vi "Read_resistance.vi"() -> ()   [LabVIEW 2017]
uses:
  <instrlib>/Agilent B2900 Series/Public/Configure/Measurement/Configure Measurement (Resistance).vi
  <instrlib>/Agilent B2900 Series/Public/Data/Read Measurement Result (Single Point).vi
  <instrlib>/Agilent B2900 Series/Agilent B2900 Series.lvlib
panel:
  out "Measurement Result":dbl
  in  "Data Mode (5: Voltage)":i32(ring)=5 items=["Current", "Resistance", "Source Output Setting", "Status", "Time", "Voltage"]
  in  "Resistance Range Lower Limit (2 Ohm)":dbl=2.0
  in  "Resistance Range Upper Limit (2E+8 Ohm)":dbl=200000000.0
  in  "Resistance NPLC (0.1)":dbl=0.1
  in  "Resistance Measurement Mode (1: Auto)":i32(ring)=1 items=["Manual", "Auto"]
  in  "Resistance Range (2 Ohm)":dbl=2.0
  in  "VISA resource name":refnum<visa-resource-name>
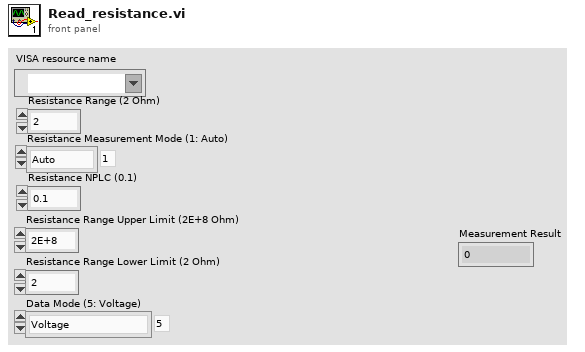
[diagram p1: front panel]
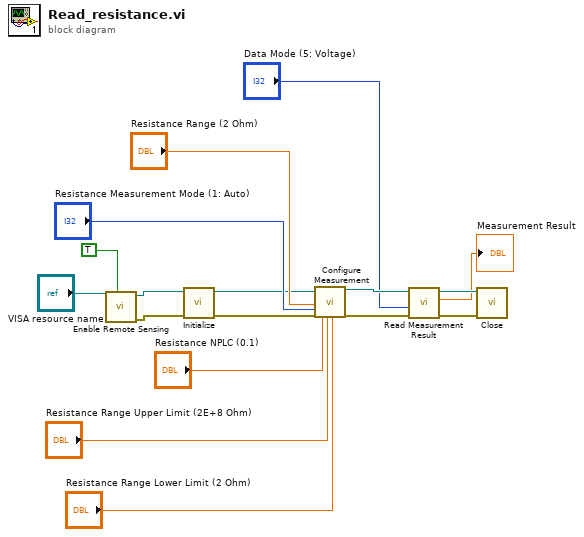
[diagram p0: block diagram]
diagram:
  n1 = call <instrlib>:"Enable Remote Sensing.vi"("Enable Remote Sensing (F: Disable)"=TRUE, "VISA resource name"="VISA resource name") -> ("error out"=w3:errorcluster, "VISA resource name out"=w1:refnum<visa-resource-name>)  [unwired: 8 in]
  n2 = call <instrlib>:"Initialize.vi"("error in (no error)"=w3, "VISA resource name"=w1) -> ("error out"=w5:errorcluster, "VISA resource name out"=w6:refnum<visa-resource-name>)  [unwired: 8 in]
  n3 = call-poly <instrlib>:"Configure Measurement.vi"("VISA resource name"=w6, "Resistance Range (2 Ohm)"="Resistance Range (2 Ohm)", "Resistance Measurement Mode (1: Auto)"="Resistance Measurement Mode (1: Auto)", "error in (no error)"=w5, "Resistance NPLC (0.1)"="Resistance NPLC (0.1)", "Resistance Range Upper Limit (2E+8 Ohm)"="Resistance Range Upper Limit (2E+8 Ohm)", "Resistance Range Lower Limit (2 Ohm)"="Resistance Range Lower Limit (2 Ohm)") -> ("VISA resource name out"=w12:refnum<visa-resource-name>, "error out"=w10:errorcluster)  [unwired: 11 in]
  n4 = call-poly <instrlib>:"Read Measurement Result.vi"("error in (no error)"=w10, "Data Mode (5: Voltage)"="Data Mode (5: Voltage)", "VISA resource name"=w12) -> ("error out"=w9:errorcluster, "Measurement Result"=→"Measurement Result":dbl, "VISA resource name out"=w11:refnum<visa-resource-name>)  [unwired: 6 in]
  n5 = call <instrlib>:"Close.vi"("error in (no error)"=w9, "VISA resource name"=w11) -> ()  [unwired: 9 in, 1 out]
